vi "ISX3_Cmd_GetSetupFrequencyList.vi"() -> (0 "get Setup Frequency List Cmd":u8[](array[numeric]))   [LabVIEW 2012, in "Sciospec ISX3 Impedance Analyzer.lvlib"]
uses:
  Sciospec ISX3 Impedance Analyzer.lvlib
panel:
  # "This VI generates the command to read the configured frequencies of a setup."
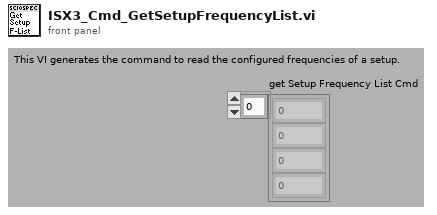
[diagram p1: front panel]
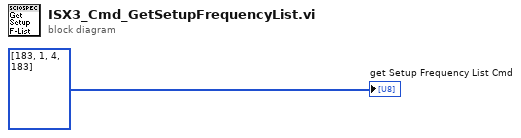
[diagram p0: block diagram]
diagram:
  "get Setup Frequency List Cmd" <- u8[] [183, 1, 4, 183]
